vi "Demo Date and Time.vi"(8 "error in (no error)":errorcluster) -> (0 "error out":errorcluster)   [LabVIEW 2011]
uses:
  VIremote.llb/VIremoteEvent.ctl
  VIremote.llb/VIremoteFunction.ctl
panel:
  in  "No properties":timestamp caption="Time Stamp" format="%<%X>T"
  out "NewVal":timestamp
  in  "Time Stamp all":timestamp caption="Time Stamp" format="%<%X\n%x>T"
  in  "UsePopup":timestamp caption="Time Stamp" format="%<%X>T"
  in  "VIremoteEvent":T1=enum."Connection Closed"
  # "Tap the Time/Date browse button above to display an iOS-date/time picker to change its value. Tapping the text field will let you edit the time as text. If you add UsePopup in the description then tapping anywhere will bring up a picker. That picker will look differently depending on the display format. For example if you only have time displayed then the picker will only let you edit the time (try below). Tapping the browse button will allways let you edit date and time.\nEditing seconds is not supported in any picker."
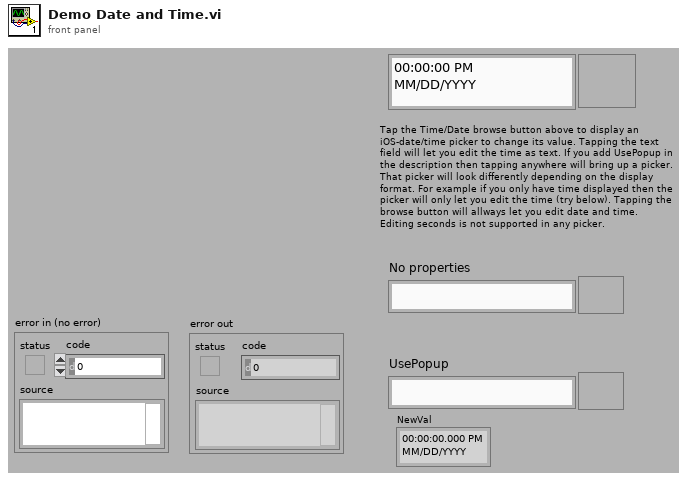
[diagram p1: front panel]
types:
  T1 = typedef "VIremoteEvent.ctl" = enum16{"No Event", "Connection Closed", "Navigate Back", "Enter Background", "Enter Foreground", "Portrait", "Portrait Upside Down", "Landscape Left", "Landscape Right"}
  T2 = typedef "VIremoteFunction.ctl" = enum16{"Do nothing", "Stop controller", "Close this connection", "Show info panel", "Set VI to control", "Set Accelerometer freq (Hz)", "Show Alert message", "Start Sound Input", "Stop Sound Input", "Set Volume (0-100)", "Set sound output Speaker", "Set sound output Receiver", "Play Sound", "Repeat Sound", "Stop Sound", "Pause Sound", "Resume Sound", "Set panel width of caller (320 or 480)", "Set Panel Size to Portrait", "Set Panel Size to Landscape", "Set Panel Size as Current Orientation", "Allow all UI Orientations", "Send user notification", "Disable Scrolling", "Normal Scrolling", "Page Scrolling", "Set Scroll Offset", "Page Indicator Position"}
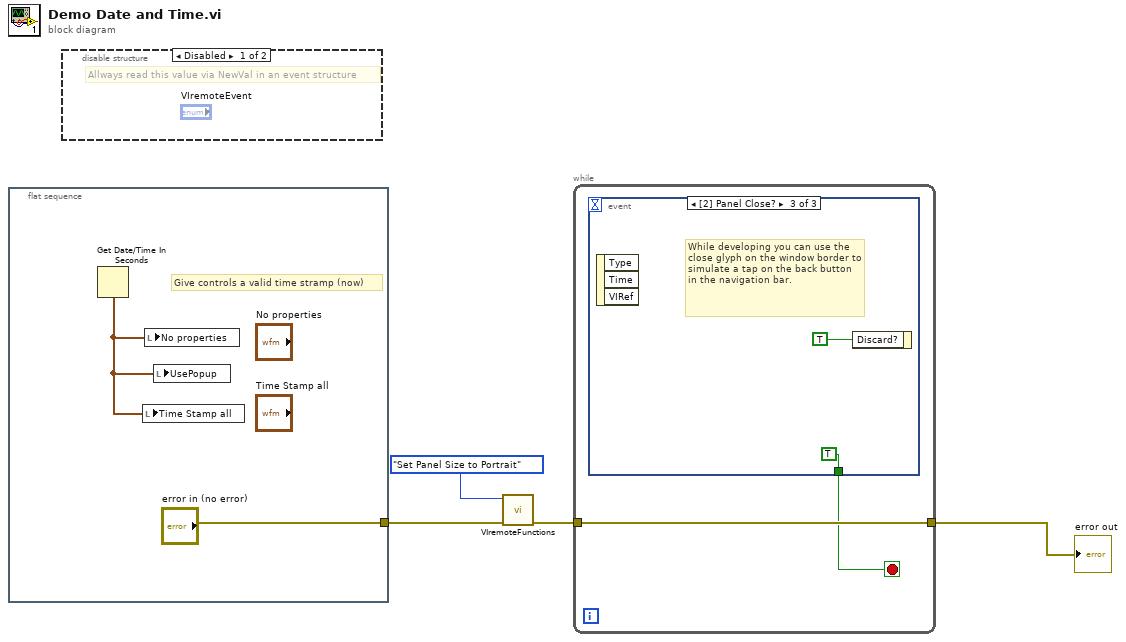
[diagram p0: block diagram]
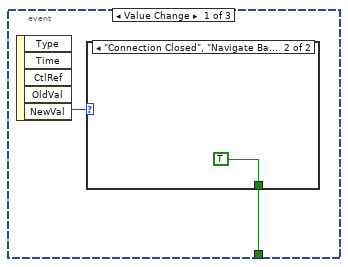
[diagram p3: hidden frame]
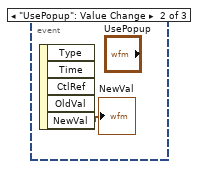
[diagram p5: hidden frame]
diagram:
  n1 = flat-sequence {
    tunnel: ["error in (no error)"] -> w2
    frame #0 {
      # "Give controls a valid time stramp (now)"
      n2 = Get Date/Time In Seconds() -> (seconds since 1Jan1904=w5:timestamp)
      n3 = local write "Time Stamp all"(w5) -> ()
      n4 = local write "No properties"(w5) -> ()
      n5 = local write "UsePopup"(w5) -> ()
    }
  }
  n6 = disable-structure shown="Disabled" {
    frame Disabled {
      # "Allways read this value via NewVal in an event structure"
    }
    frame Enabled {
    }
  }
  n7 = call "VIremoteFunctions.vi"("error in (no error)"=w2, "Function"=VIremoteFunction."Set Panel Size to Portrait") -> ("error out"=w3:errorcluster)  [unwired: 4 in, 5 out]
  n8 = while {
    tunnel: [w8] -> w1
    tunnel: w3 -> [w8]
    stop <- w7 stop-if-true
    n9 = event shown="[2] Panel Close?" {
      selector: _ -> [_ _ _]
      dyn-events: _ -> [_ _ _]
      timeout: _ -> [_ _ _]
      tunnel: [w9 _ TRUE] -> w7
      event Value Change {
        n10 = event-data() -> ("NewVal"=w10:T1)  [unwired: 5 out]
        n11 = case shown="\"Connection Closed\", \"Navigate Back\"" w10 {
          tunnel: [_ TRUE] -> w9
          frame "No Event", Default {
          }
          frame "Connection Closed", "Navigate Back" {
          }
        }
      }
      event "UsePopup": Value Change {
        n12 = event-data() -> ("NewVal"=→"NewVal":timestamp)  [unwired: 5 out]
      }
      event Panel Close? {
        # "While developing you can use the close glyph on the window border to simulate a tap on the back button in the navigation bar."
        n13 = event-data() -> ()  [unwired: 4 out]
        n14 = event-data("Discard?"=TRUE) -> ()  [unwired: 1 in, 1 out]
      }
    }
  }
  "error out" <- w1
